vi "RegisterForEvents.vi"(8 "error in (no error)":errorcluster, 11 "EventTestListener in":refnum<class "EventTestListener.lvclass">) -> (0 "error out":errorcluster, 2 "Event Registration Refnum":refnum<event-registration>, 3 "EventTestListener out":refnum<class "EventTestListener.lvclass">)   [LabVIEW 2019, in "TestExplorer.lvlib" / "EventTestListener.lvclass"]
uses:
  EventTestListener.lvclass
  TestCase/TestCase/TestCase.lvclass
  FailureEventData.ctl
  TestEndedEventData.ctl
  TestSuite/TestSuite.lvclass
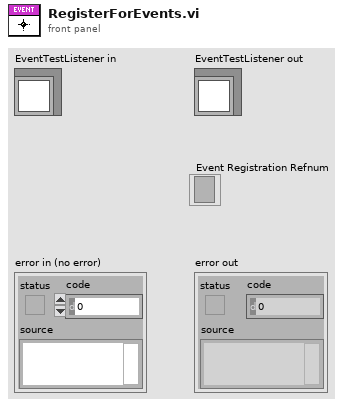
[diagram p1: front panel]
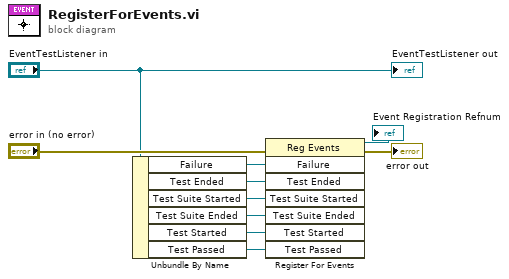
[diagram p0: block diagram]
diagram:
  n1 = Unbundle By Name("EventTestListener in") -> ("Failure"=w7:refnum<user-event>, "Test Ended"=w6:refnum<user-event>, "Test Suite Started"=w5:refnum<user-event>, "Test Suite Ended"=w4:refnum<user-event>, "Test Started"=w3:refnum<user-event>, "Test Passed"=w2:refnum<user-event>)
  n2 = register-events(error in="error in (no error)", w7, w6, w5, w4, w3, w2) -> (reference out=→"Event Registration Refnum":refnum<event-registration>, error out=→"error out":errorcluster)  [unwired: 1 in]
  "EventTestListener out" <- "EventTestListener in"
